vi "subMFD_Filter Coef.vi"(11 "h(n)":dbl[](array[numeric]) format="%#_10g") -> (3 "Coefficients Report":string)   [LabVIEW 2023]
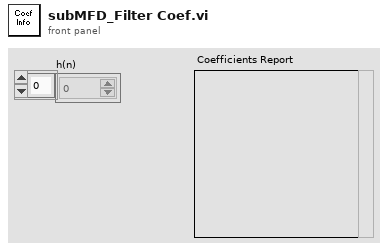
[diagram p1: front panel]
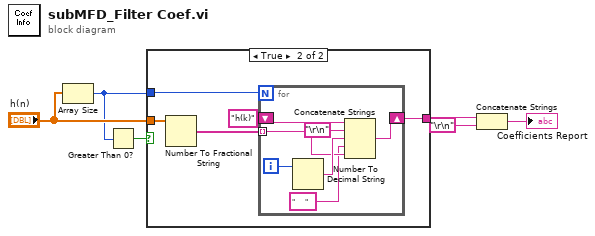
[diagram p0: block diagram]
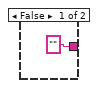
[diagram p2: hidden frame]
diagram:
  n1 = Array Size(array="h(n)") -> (size(s)=w4:i32)
  n2 = Greater Than 0?(x=w4) -> (x > 0?=w5:bool)
  n3 = case shown="True" w5 {
    tunnel: "h(n)" -> [_ w11]
    tunnel: w4 -> [_ w9]
    tunnel: ["" ("Coefficients Report") w8] -> w3
    frame False {
    }
    frame True {
      n4 = Number To Fractional String(number=w11) -> (F-format string=w10:string[])  [unwired: 3 out]
      n5 = for {
        N: w9 -> [_]
        shift-right: [w19] -> w8
        shift-left: "h(k)" ("Coefficients Report") -> [w18]
        tunnel: w10 -> [w14] mode=indexing
        i -> [w16]
        n6 = Number To Decimal String(number=w16) -> (decimal integer string=w15:string)  [unwired: 1 out]
        n7 = Concatenate Strings(w18, "\r\n", w15, "     ", w14) -> (w19:string)
      }
    }
  }
  n8 = Concatenate Strings(w3, "\r\n") -> (→"Coefficients Report":string)
